vi "ELEV_SET_STATE.vi"(10 "argv":string[](array[string]), 11 "args":u8) -> ()   [LabVIEW 2011]
panel:
  in  "StateMaps":T1(array[cluster])=[{"Name"="floor", "State"=enum."Floor"}, {"Name"="carry", "State"=enum."Carry"}, {"Name"="score_low", "State"=enum."Score LOW"}, {"Name"="score_mid", "State"=enum."Score MID"}, {"Name"="score_hi", "State"=enum."Score HI"}, {"Name"="b_slot", "State"=enum."B-Slot"}]
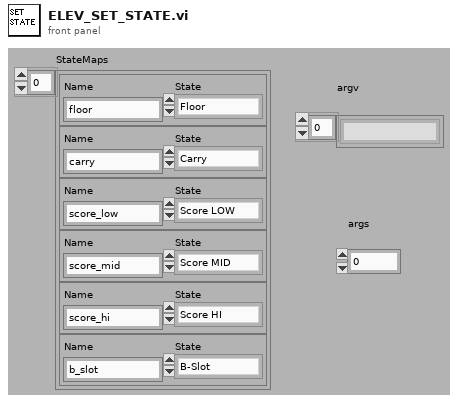
[diagram p1: front panel]
types:
  T1 = cluster{"Name":string, "State":enum16{"B-Wall", "Wall", "B-Slot", "Slot", "Fold", "Carry", "Floor", "Score LOW", "Score MID", "Score HI"}}[]
  T2 = enum16{"B-Wall", "Wall", "B-Slot", "Slot", "Fold", "Carry", "Floor", "Score LOW", "Score MID", "Score HI"}
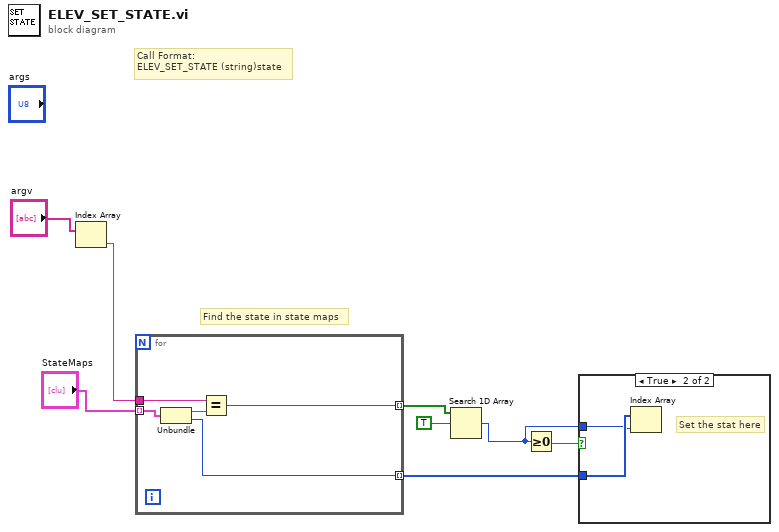
[diagram p0: block diagram]
diagram:
  # "Find the state in state maps"
  # "Call Format:\nELEV_SET_STATE (string)state"
  n1 = Index Array(array="argv") -> (element=w7:string)  [unwired: 1 in]
  n2 = for {
    tunnel: w7 -> [w13]
    tunnel: "StateMaps" -> [w12] mode=indexing
    tunnel: [w10] -> w5 mode=indexing
    tunnel: [w9] -> w2 mode=indexing
    n3 = Unbundle(w12) -> ("Name"=w11:string, "State"=w9:T2)
    n4 = Equal?(x=w13, y=w11) -> (x = y?=w10:bool)
  }
  n5 = Search 1D Array(1D array=w5, element=TRUE) -> (index of element=w1:i32)  [unwired: 1 out]
  n6 = Greater Or Equal To 0?(x=w1) -> (x >= 0?=w3:bool)
  n7 = case shown="True" w3 {
    tunnel: w2 -> [_ w15]
    tunnel: w1 -> [_ w14]
    frame False {
    }
    frame True {
      # "Set the stat here"
      n8 = Index Array(array=w15, index=w14) -> ()  [unwired: 1 out]
    }
  }
